vi "IsValueChange.vi"(1 "Variant":variant) -> (0 "result":bool)   [LabVIEW 2015]
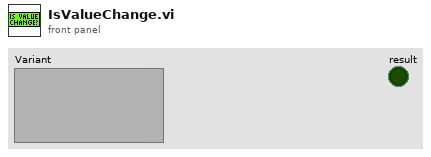
[diagram p1: front panel]
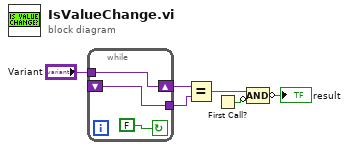
[diagram p0: block diagram]
diagram:
  n1 = while {
    tunnel: "Variant" -> [w9]
    shift-right: [w9] -> w5
    shift-left: _ -> [w8]
    tunnel: [w8] -> w4
    stop <- FALSE continue-if-true
  }
  n2 = Equal?(x=w5, y=w4) -> (x = y?=w3:bool)
  n3 = First Call?() -> (First Call?: T/F=w2:bool)
  n4 = Compound Arithmetic op=AND(w3, invert w2) -> (invert →"result":bool)
